vi "shared memory write.vi"(6 "channel classification":T1, 8 "error in":errorcluster, 10 "data table":T2, 11 "module in":refnum<class "Shared Memory Runtime.lvclass">) -> (0 "error out":errorcluster, 2 "data table out":T2, 3 "module out":refnum<class "Shared Memory Runtime.lvclass">)   [LabVIEW 2013, in "Shared Memory Runtime.lvclass"]
uses:
  Shared Memory Runtime.lvclass
  <vilib>/NI/Tag Bus/table/data table.ctl
  <vilib>/NI/Tag Bus Module Framework/channel/channel classification.ctl
  <vilib>/NI/Tag Bus/table/data polymorphs/read many/read Doubles.vi
  <vilib>/NI/Tag Bus/table/data polymorphs/read many/read Singles.vi
  <vilib>/NI/Tag Bus/table/data polymorphs/read many/read I64s.vi
  <vilib>/NI/Tag Bus/table/data polymorphs/read many/read I32s.vi
  <vilib>/NI/Tag Bus/table/data polymorphs/read many/read I16s.vi
  <vilib>/NI/Tag Bus/table/data polymorphs/read many/read I8s.vi
  <vilib>/NI/Tag Bus/table/data polymorphs/read many/read U64s.vi
  <vilib>/NI/Tag Bus/table/data polymorphs/read many/read U32s.vi
  <vilib>/NI/Tag Bus/table/data polymorphs/read many/read U16s.vi
  <vilib>/NI/Tag Bus/table/data polymorphs/read many/read U8s.vi
  <vilib>/NI/Tag Bus/table/data polymorphs/read many/read Booleans.vi
  <vilib>/National Instruments/Shared Memory Library for Linux RT/VIs/Miscellaneous/Get Shared Object Path.vi
  <vilib>/Utility/libraryn.llb/Check if File or Folder Exists.vi
  <vilib>/Utility/error.llb/Error Cluster From Error Code.vi
  <vilib>/NI/Tag Bus/table/data table.lvlib
  <vilib>/National Instruments/Shared Memory Library for Linux RT/Shared Memory.lvlib
  <vilib>/NI/Tag Bus Module Framework/channel/TBM channel.lvclass
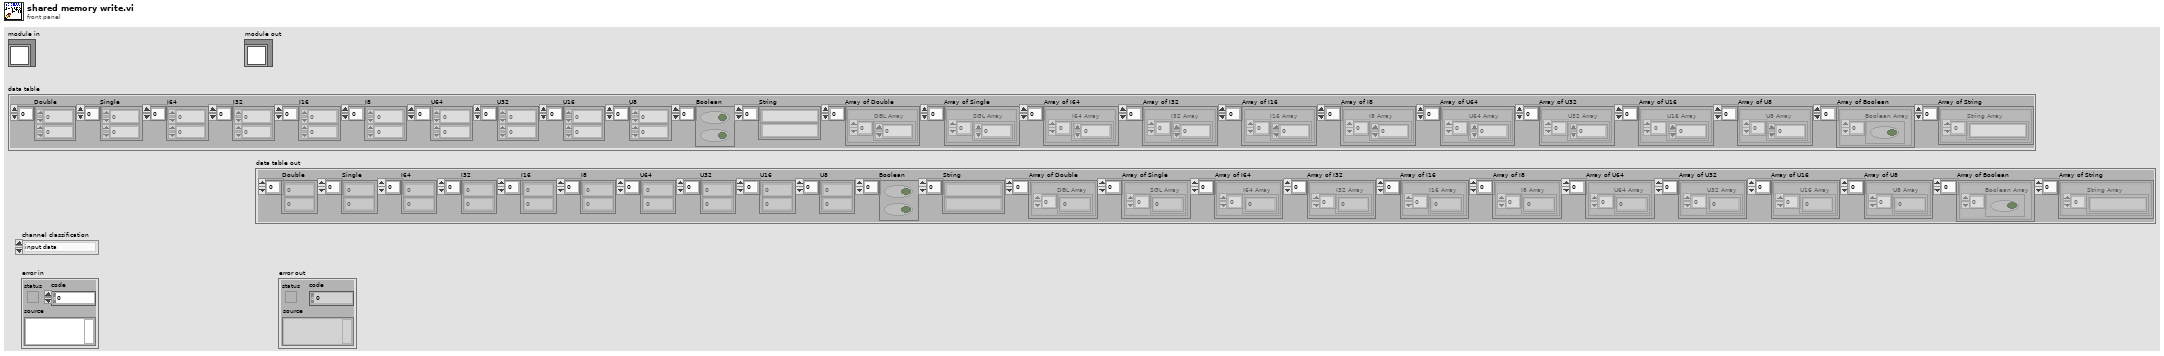
[diagram p1: front panel]
types:
  T1 = typedef "TBM channel.lvclass/channel classification.ctl" = enum16{"input data", "output data", "processing parameter", "processing result"}
  T2 = typedef "tag bus.lvlib/data table.lvlib/data table.ctl" = cluster{"Double":dbl[], "Single":sgl[], "I64":i64[], "I32":i32[], "I16":i16[], "I8":i8[], "U64":u64[], "U32":u32[], "U16":u16[], "U8":u8[], "Boolean":bool[], "String":string[], "Array of Double":cluster{"DBL Array":dbl[]}[], "Array of Single":cluster{"SGL Array":sgl[]}[], "Array of I64":cluster{"I64 Array":i64[]}[], "Array of I32":cluster{"I32 Array":i32[]}[], "Array of I16":cluster{"I16 Array":i16[]}[], "Array of I8":cluster{"I8 Array":i8[]}[], "Array of U64":cluster{"U64 Array":u64[]}[], "Array of U32":cluster{"U32 Array":u32[]}[], "Array of U16":cluster{"U16 Array":u16[]}[], "Array of U8":cluster{"U8 Array":u8[]}[], "Array of Boolean":cluster{"Boolean Array":bool[]}[], "Array of String":cluster{"String Array":string[]}[]}
  T3 = typedef "shared memory runtime.lvclass/shared memory module runtime.ctl" = cluster{"channel classification":T1, "data type":T4, "pointer to shared memory":u64, "number of elements":u64, "data dictionary index":cluster{i32[]}, "shared memory":T5}
  T4 = typedef "tag bus.lvlib/tag descriptor.lvclass/Data Type.ctl" = enum16{"Double", "Single", "I64", "I32", "I16", "I8", "U64", "U32", "U16", "U8", "Boolean", "String", "Array of Double", "Array of Single", "Array of I64", "Array of I32", "Array of I16", "Array of I8", "Array of U64", "Array of U32", "Array of U16", "Array of U8", "Array of Boolean", "Array of String"}
  T5 = typedef "Shared Memory Class Reference.ctl" = refnum<data-value>
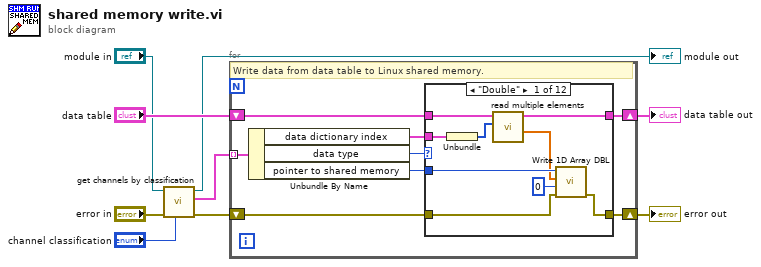
[diagram p0: block diagram]
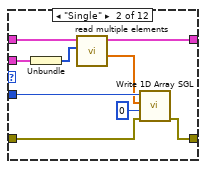
[diagram p2: hidden frame]
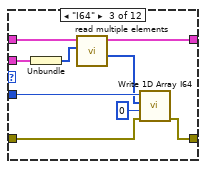
[diagram p3: hidden frame]
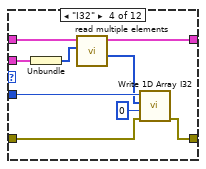
[diagram p4: hidden frame]
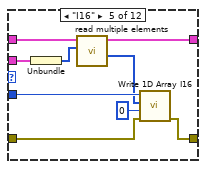
[diagram p5: hidden frame]
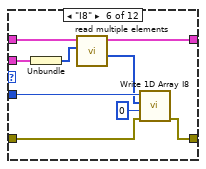
[diagram p6: hidden frame]
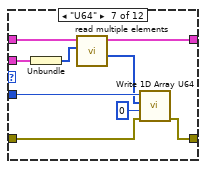
[diagram p7: hidden frame]
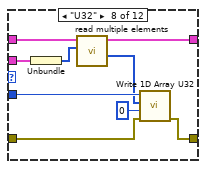
[diagram p8: hidden frame]
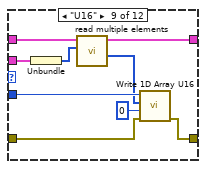
[diagram p9: hidden frame]
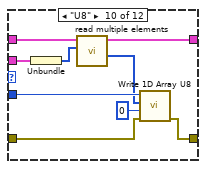
[diagram p10: hidden frame]
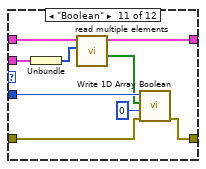
[diagram p11: hidden frame]
diagram:
  n1 = call "get channels by classification.vi"("channel classification"="channel classification", "error in"="error in", "shared memory runtime in"="module in") -> ("error out"=w5:errorcluster, "channels"=w4:T3[], "shared memory runtime out"=→"module out":refnum<class "Shared Memory Runtime.lvclass">)  [unwired: 6 in]
  n2 = for {
    tunnel: w4 -> [w15] mode=indexing
    shift-right: [w11] -> w8
    shift-left: w5 -> [w12]
    shift-right: [w17] -> w2
    shift-left: "data table" -> [w16]
    # "Write data from data table to Linux shared memory."
    n3 = Unbundle By Name(w15) -> ("data dictionary index"=w10:cluster{i32[]}, "data type"=w13:T4, "pointer to shared memory"=w14:u64)
    n4 = case shown="\"Double\"" w13 {
      tunnel: w16 -> [w26 w35 w44 w53 w62 w71 w80 w89 w98 w107 w116 w118]
      tunnel: [w25 w34 w43 w52 w61 w70 w79 w88 w97 w106 w115 w118] -> w17
      tunnel: w12 -> [w20 w29 w38 w47 w56 w65 w74 w83 w92 w101 w110 w117]
      tunnel: [w19 w28 w37 w46 w55 w64 w73 w82 w91 w100 w109 w117] -> w11
      tunnel: w14 -> [w21 w30 w39 w48 w57 w66 w75 w84 w93 w102 w111 _]
      tunnel: w10 -> [w24 w33 w42 w51 w60 w69 w78 w87 w96 w105 w114 _]
      frame "Double" {
        n5 = Unbundle(w24) -> (w23:i32[])
        n6 = call-poly <vilib>:"read multiple elements.vi"("indices"=w23, "data table in"=w26) -> ("values"=w18:dbl[], "data table out"=w25:T2)  [unwired: 8 in]
        n7 = call <vilib>:"Write 1D Array DBL.vi"("error in (no error)"=w20, "start index"=u64 0, "value"=w18, "pointer"=w21) -> ("error out"=w19:errorcluster)  [unwired: 4 in, 3 out]
      }
      frame "Single" {
        n8 = Unbundle(w33) -> (w32:i32[])
        n9 = call-poly <vilib>:"read multiple elements.vi"("indices"=w32, "data table in"=w35) -> ("values"=w27:sgl[], "data table out"=w34:T2)  [unwired: 8 in]
        n10 = call <vilib>:"Write 1D Array SGL.vi"("error in (no error)"=w29, "start index"=u64 0, "value"=w27, "pointer"=w30) -> ("error out"=w28:errorcluster)  [unwired: 4 in, 3 out]
      }
      frame "I64" {
        n11 = Unbundle(w42) -> (w41:i32[])
        n12 = call-poly <vilib>:"read multiple elements.vi"("indices"=w41, "data table in"=w44) -> ("values"=w36:i64[], "data table out"=w43:T2)  [unwired: 8 in]
        n13 = call <vilib>:"Write 1D Array I64.vi"("error in (no error)"=w38, "start index"=u64 0, "value"=w36, "pointer"=w39) -> ("error out"=w37:errorcluster)  [unwired: 4 in, 3 out]
      }
      frame "I32" {
        n14 = Unbundle(w51) -> (w50:i32[])
        n15 = call-poly <vilib>:"read multiple elements.vi"("indices"=w50, "data table in"=w53) -> ("values"=w45:i32[], "data table out"=w52:T2)  [unwired: 8 in]
        n16 = call <vilib>:"Write 1D Array I32.vi"("error in (no error)"=w47, "start index"=u64 0, "value"=w45, "pointer"=w48) -> ("error out"=w46:errorcluster)  [unwired: 4 in, 3 out]
      }
      frame "I16" {
        n17 = Unbundle(w60) -> (w59:i32[])
        n18 = call-poly <vilib>:"read multiple elements.vi"("indices"=w59, "data table in"=w62) -> ("values"=w54:i16[], "data table out"=w61:T2)  [unwired: 8 in]
        n19 = call <vilib>:"Write 1D Array I16.vi"("error in (no error)"=w56, "start index"=u64 0, "value"=w54, "pointer"=w57) -> ("error out"=w55:errorcluster)  [unwired: 4 in, 3 out]
      }
      frame "I8" {
        n20 = Unbundle(w69) -> (w68:i32[])
        n21 = call-poly <vilib>:"read multiple elements.vi"("indices"=w68, "data table in"=w71) -> ("values"=w63:i8[], "data table out"=w70:T2)  [unwired: 8 in]
        n22 = call <vilib>:"Write 1D Array I8.vi"("error in (no error)"=w65, "start index"=u64 0, "value"=w63, "pointer"=w66) -> ("error out"=w64:errorcluster)  [unwired: 4 in, 3 out]
      }
      frame "U64" {
        n23 = Unbundle(w78) -> (w77:i32[])
        n24 = call-poly <vilib>:"read multiple elements.vi"("indices"=w77, "data table in"=w80) -> ("values"=w72:u64[], "data table out"=w79:T2)  [unwired: 8 in]
        n25 = call <vilib>:"Write 1D Array U64.vi"("error in (no error)"=w74, "start index"=u64 0, "value"=w72, "pointer"=w75) -> ("error out"=w73:errorcluster)  [unwired: 4 in, 3 out]
      }
      frame "U32" {
        n26 = Unbundle(w87) -> (w86:i32[])
        n27 = call-poly <vilib>:"read multiple elements.vi"("indices"=w86, "data table in"=w89) -> ("values"=w81:u32[], "data table out"=w88:T2)  [unwired: 8 in]
        n28 = call <vilib>:"Write 1D Array U32.vi"("error in (no error)"=w83, "start index"=u64 0, "value"=w81, "pointer"=w84) -> ("error out"=w82:errorcluster)  [unwired: 4 in, 3 out]
      }
      frame "U16" {
        n29 = Unbundle(w96) -> (w95:i32[])
        n30 = call-poly <vilib>:"read multiple elements.vi"("indices"=w95, "data table in"=w98) -> ("values"=w90:u16[], "data table out"=w97:T2)  [unwired: 8 in]
        n31 = call <vilib>:"Write 1D Array U16.vi"("error in (no error)"=w92, "start index"=u64 0, "value"=w90, "pointer"=w93) -> ("error out"=w91:errorcluster)  [unwired: 4 in, 3 out]
      }
      frame "U8" {
        n32 = Unbundle(w105) -> (w104:i32[])
        n33 = call-poly <vilib>:"read multiple elements.vi"("indices"=w104, "data table in"=w107) -> ("values"=w99:u8[], "data table out"=w106:T2)  [unwired: 8 in]
        n34 = call <vilib>:"Write 1D Array U8.vi"("error in (no error)"=w101, "start index"=u64 0, "value"=w99, "pointer"=w102) -> ("error out"=w100:errorcluster)  [unwired: 4 in, 3 out]
      }
      frame "Boolean" {
        n35 = Unbundle(w114) -> (w113:i32[])
        n36 = call-poly <vilib>:"read multiple elements.vi"("indices"=w113, "data table in"=w116) -> ("values"=w108:bool[], "data table out"=w115:T2)  [unwired: 8 in]
        n37 = call <vilib>:"Write 1D Array Boolean.vi"("error in (no error)"=w110, "start index"=u64 0, "value"=w108, "pointer"=w111) -> ("error out"=w109:errorcluster)  [unwired: 4 in, 3 out]
      }
      frame Default {
      }
    }
  }
  "error out" <- w8
  "data table out" <- w2
